vi "Run Tests.vi"() -> ()   [LabVIEW 2013]
panel:
  out "Results":T1(array[cluster])
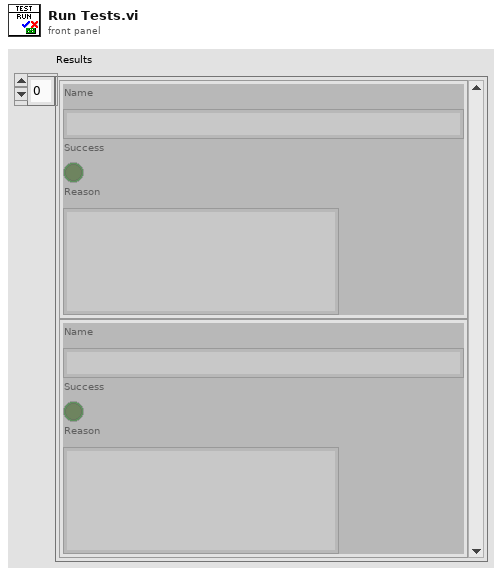
[diagram p1: front panel]
types:
  T1 = cluster{"Name":string, "Success":bool, "Reason":string}[]
  T2 = cluster{"Name":string, "Success":bool, "Reason":string}
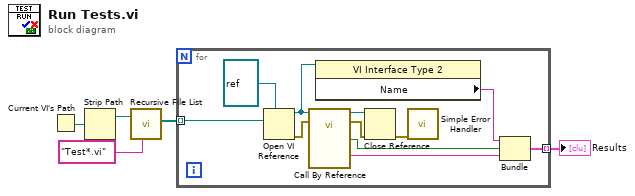
[diagram p0: block diagram]
diagram:
  n1 = Current VI's Path() -> (path=w5:path)
  n2 = Strip Path(path=w5) -> (stripped path=w4:path)  [unwired: 1 out]
  n3 = call <vilib>:"Recursive File List.vi"("pattern"="Test*.vi", "Folder Path"=w4) -> ("All Files in Dir"=w2:path[])  [unwired: 5 in, 4 out]
  n4 = for {
    tunnel: w2 -> [w11] mode=indexing
    tunnel: [w6] -> w1 mode=indexing
    n5 = Open VI Reference(type specifier VI Refnum (for type only)=refnum<vi> refnum, vi path=w11) -> (vi reference=w10:refnum<vi>, error out=w15:errorcluster)  [unwired: 4 in]
    n6 = call-by-ref "?"(reference=w10, error in=w15) -> (reference out=w14:refnum<vi>, error out=w13:errorcluster, "Reason"=w7:string, "Success"=w8:bool)
    n7 = property class="VI Interface Type 2"(reference=w10) -> ("Name"=w9:string)  [unwired: 1 in, 2 out]
    n8 = Close Reference(reference=w14, error in (no error)=w13) -> (error out=w12:errorcluster)
    n9 = call <vilib>:"Simple Error Handler.vi"("error in (no error)"=w12) -> ()  [unwired: 4 in, 5 out]
    n10 = Bundle("Name"=w9, "Success"=w8, "Reason"=w7) -> (w6:T2)  [unwired: 1 in]
  }
  "Results" <- w1
